vi "BasicUsage.vi"() -> ()   [LabVIEW 2023, in "Examples.lvlib"]
uses:
  Examples.lvlib
  Classes/DeviceManager/DeviceManager.lvlib
panel:
  out "error out":errorcluster
  in  "error in":errorcluster
  # "See Block Diagram for explanation..."
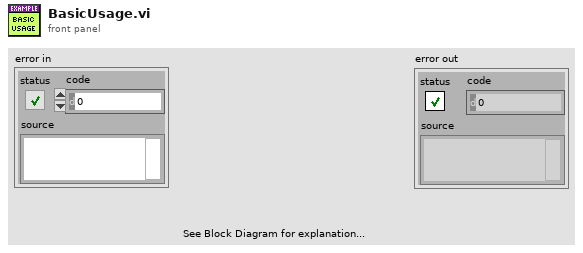
[diagram p1: front panel]
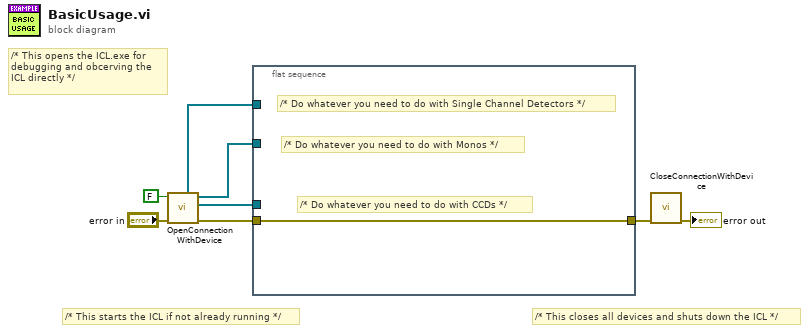
[diagram p0: block diagram]
diagram:
  # "/* This opens the ICL.exe for\ndebugging and obcerving the\nICL directly */"
  # "/* This closes all devices and shuts down the ICL */"
  # "/* This starts the ICL if not already running */"
  n1 = call "OpenConnectionWithDevice.vi"("error in"="error in", "show ICL for debugging"=FALSE) -> ("error out"=w5:errorcluster, "CCDs"=w6:refnum<class "CCD.lvclass">[], "Monos"=w7:refnum<class "Monochromator.lvclass">[], "SCDs"=w8:refnum<class "SCD.lvclass">[])  [unwired: 5 in, 1 out]
  n2 = flat-sequence {
    tunnel: w8 -> [_]
    tunnel: w7 -> [_]
    tunnel: w6 -> [_]
    tunnel: w5 -> [w9]
    tunnel: [w9] -> w4
    frame #0 {
      # "/* Do whatever you need to do with CCDs */"
      # "/* Do whatever you need to do with Monos */"
      # "/* Do whatever you need to do with Single Channel Detectors */"
    }
  }
  n3 = call "CloseConnectionWithDevice.vi"("error in (no error)"=w4) -> ("error out"=→"error out":errorcluster)  [unwired: 10 in]
